vi "OC2 Read status.vi"(0 "VISA resource name":refnum<visa-resource-name>, 1 "enable":bool, 2 "feedback read buffer":string, 3 "error in":errorcluster) -> (4 "RX packet ok":bool, 5 "dup VISA resource name":refnum<visa-resource-name>, 6 "feedback buffer":string, 7 "Report cluster":T1, 8 "error out":errorcluster)   [LabVIEW 2009]
doc: "TCM Read Alarm.vi\n\nVI that reads status report information, accepts a cluster that contains the following variables:\nSetpoint - current setpoint value\nTemperature - Current temperature from TCM\nControl - state of the control\nOutput - current output % value\nAlarms - state of the alarms\nFaults - fault indicator\nTemp 0k. - Temperature within limits\nSupply vdc - TCM current supply voltage\nVersion - Firmware version\nTest Cycle - current test cycle\nTest Mode - current test mode\n\nCOPYRIGHT ELECTRON DYNAMICS LTD"
panel:
  in  "Command":string="j"
  in  "Min Expected no \nof characters":u32=54
  # "Read status report"
  # "V1.02"
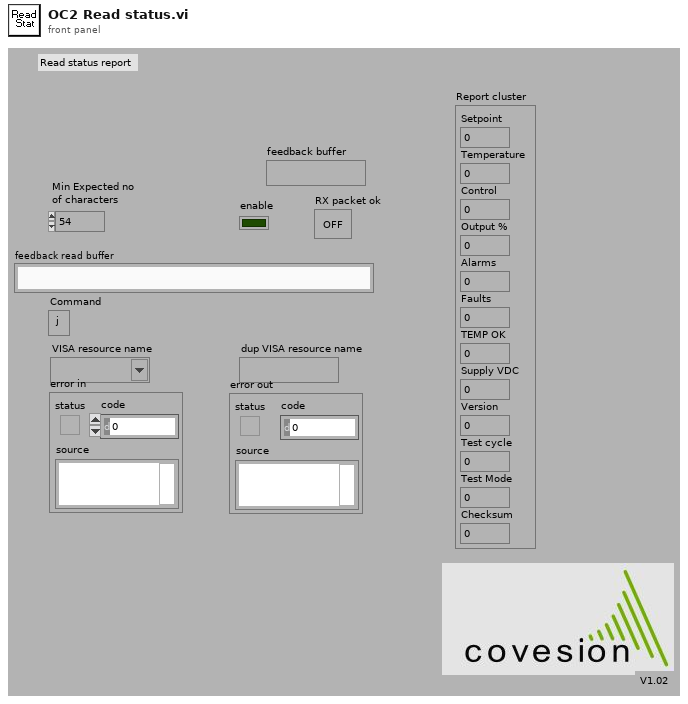
[diagram p1: front panel]
types:
  T1 = cluster{"Setpoint":dbl, "Temperature":dbl, "Control":i32, "Output %":dbl, "Alarms":i32, "Faults":i32, "TEMP OK":i32, "Supply VDC":dbl, "Version":dbl, "Test cycle":i32, "Test Mode":i32, "Checksum":i32}
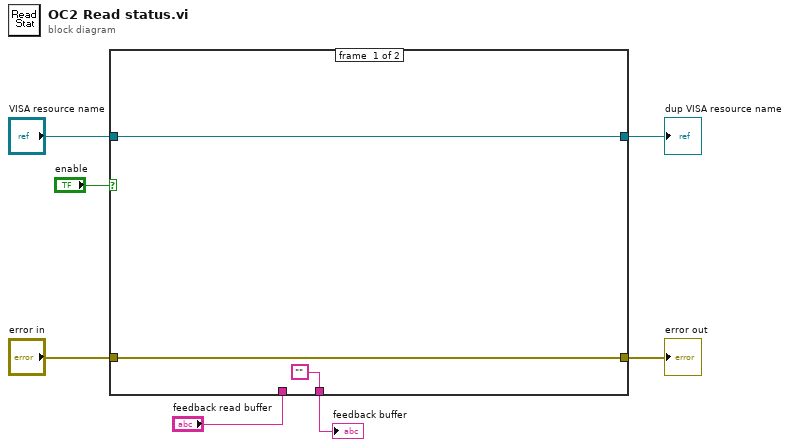
[diagram p0: block diagram]
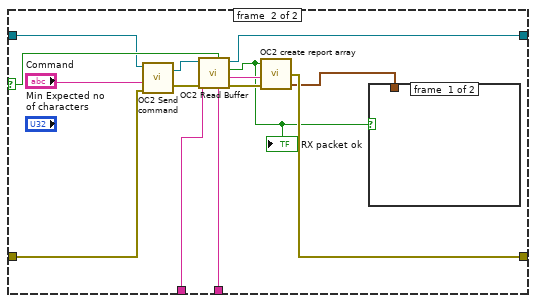
[diagram p2: hidden frame]
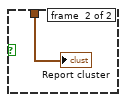
[diagram p3: hidden frame]
diagram:
  n1 = case shown="True" "enable" {
    selector: "enable" -> [_ w21]
    tunnel: "VISA resource name" -> [w10 w18]
    tunnel: [w10 w24] -> w6
    tunnel: "error in" -> [w9 w16]
    tunnel: [w9 w13] -> w4
    tunnel: "feedback read buffer" -> [_ w23]
    tunnel: ["" w22] -> w2
    frame #0 {
    }
    frame #1 {
      n2 = call "OC2 Send command.vi"("VISA resource name"=w18, "Command"="Command", "error in (no error)"=w16) -> ("dup VISA resource name"=w19:refnum<visa-resource-name>, "error out"=w20:errorcluster)  [unwired: 2 in]
      n3 = call "OC2 Read Buffer.vi"("COMS IN"=w21, "error in (no error)"=w20, "fedback read buffer"=w23, "VISA resource name"=w19) -> ("error out"=w15:errorcluster, "Report string"=w14:string, "RX packet ok"=w12:bool, "VISA resource name out"=w24:refnum<visa-resource-name>, "feedback buffer"=w22:string)  [unwired: 3 in]
      "RX packet ok" <- w12
      n4 = call "OC2 create report array.vi"("error in"=w15, "report string"=w14, "rx packet ok"=w12) -> ("Report cluster"=w11:T1, "error out"=w13:errorcluster)  [unwired: 1 in]
      n5 = case shown="True" w12 {
        tunnel: w11 -> [_ w25]
        frame #0 {
        }
        frame #1 {
          "Report cluster" <- w25
        }
      }
    }
  }
  "dup VISA resource name" <- w6
  "error out" <- w4
  "feedback buffer" <- w2
